vi "goToStandby.vi"(8 "error in (no error)":errorcluster, 10 "model":refnum<class "Model.lvclass">, 11 "EnabledState in":refnum<class "EnabledState.lvclass">) -> (0 "error out":errorcluster, 2 "model 2":refnum<class "Model.lvclass">, 3 "EnabledState out":refnum<class "EnabledState.lvclass">)   [LabVIEW 2013, in "EnabledState.lvclass"]
uses:
  EnabledState.lvclass
  Model/Model/Model.lvclass
  Typedefs/StateSelector.ctl
  Typedefs/AITDTTypedefs.lvlib
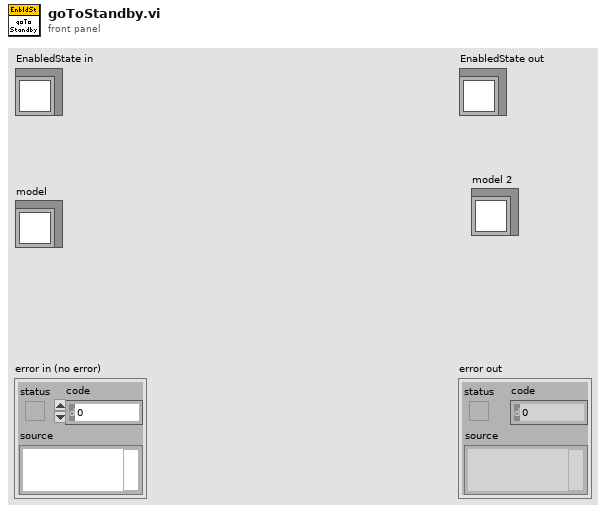
[diagram p1: front panel]
types:
  T1 = typedef "AITDTTypedefs.lvlib/StateSelector.ctl" = enum16{"AwaitingSetpointAcknowledgmentState", "EndingCycleState", "FaultState", "OffState", "PausingState", "RequestingNewSetpointState", "SamplingState", "SettlingState", "SoakingState", "StabilizingState", "StandbyState", "StoppedState", "TransitioningTemperatureState"}
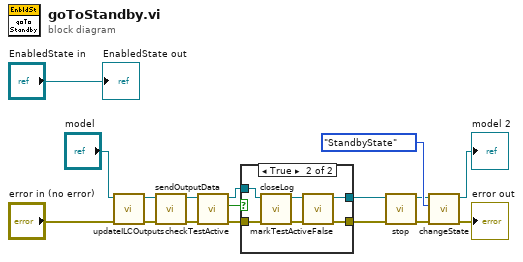
[diagram p0: block diagram]
diagram:
  n1 = call "updateILCOutputs.vi"("error in (no error)"="error in (no error)", "Model in"="model") -> ("error out"=w9:errorcluster, "Model out"=w10:refnum<class "Model.lvclass">)  [unwired: 8 in]
  n2 = call "sendOutputData.vi"("error in (no error)"=w9, "Model in"=w10) -> ("error out"=w7:errorcluster, "Model out"=w8:refnum<class "Model.lvclass">)  [unwired: 8 in]
  n3 = call "checkTestActive.vi"("error in (no error)"=w7, "Model in"=w8) -> ("error out"=w11:errorcluster, "testActiveIsTrue"=w13:bool, "Model out"=w12:refnum<class "Model.lvclass">)  [unwired: 7 in]
  n4 = case shown="True" w13 {
    tunnel: [w19 w22] -> w6
    tunnel: [w18 w20] -> w4
    tunnel: w12 -> [w19 w25]
    tunnel: w11 -> [w18 w24]
    frame False {
    }
    frame True {
      n5 = call "closeLog.vi"("error in (no error)"=w24, "Model in"=w25) -> ("error out"=w21:errorcluster, "Model out"=w23:refnum<class "Model.lvclass">)  [unwired: 8 in]
      n6 = call "markTestActiveFalse.vi"("error in (no error)"=w21, "Model in"=w23) -> ("error out"=w20:errorcluster, "Model out"=w22:refnum<class "Model.lvclass">)  [unwired: 8 in]
    }
  }
  n7 = call "stop.vi"("error in (no error)"=w4, "Model in"=w6) -> ("error out"=w3:errorcluster, "Model out"=w5:refnum<class "Model.lvclass">)  [unwired: 8 in]
  n8 = call "changeState.vi"("error in (no error)"=w3, "State:"=StateSelector."StandbyState", "Model in"=w5) -> ("error out"=→"error out":errorcluster, "Model out"=→"model 2":refnum<class "Model.lvclass">)  [unwired: 7 in]
  "EnabledState out" <- "EnabledState in"
